vi "Write Loop order.vi"(10 "Loop order":bool, 11 "Toggle 8 in":refnum<class "Toggle 8.lvclass">) -> (3 "Toggle 8 out":refnum<class "Toggle 8.lvclass">)   [LabVIEW 2020, in "Toggle 8.lvclass"]
uses:
  Toggle 8.lvclass
  Toggle 8.lvclass/Toggle 8.ctl
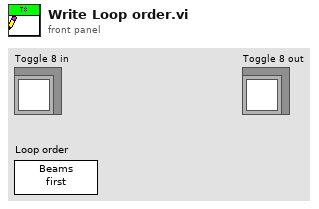
[diagram p1: front panel]
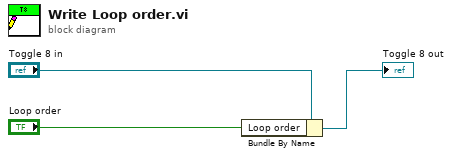
[diagram p0: block diagram]
diagram:
  n1 = Bundle By Name(cluster="Toggle 8 in", "Loop order"="Loop order") -> (→"Toggle 8 out":refnum<class "Toggle 8.lvclass">)
